vi "COPY_DLL_TO_C.vi"(8 "error in (no error)":errorcluster, 10 "appended path in":path) -> (0 "error out":errorcluster, 2 "appended path out":path)   [LabVIEW 2015, in "VIS-NIR.lvclass"]
uses:
  VIS-IR/VIS-NIR.lvclass
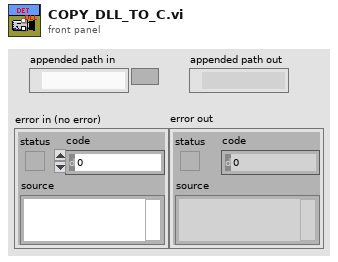
[diagram p1: front panel]
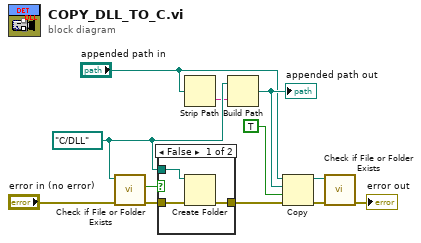
[diagram p0: block diagram]
diagram:
  w10 = path "C:/DLL" ("appended path")
  n1 = call <vilib>:"Check if File or Folder Exists.vi"("error in (no error)"="error in (no error)", "path"=w10) -> ("error out"=w9:errorcluster, "file or folder exists?"=w7:bool)  [unwired: 7 in, 1 out]
  n2 = case shown="False" w7 {
    tunnel: [w13 w16] -> w8
    tunnel: w9 -> [w14 w16]
    tunnel: w10 -> [w15 _]
    frame False {
      n3 = Create Folder(path (use dialog)=w15, error in=w14) -> (error out=w13:errorcluster)  [unwired: 1 in, 2 out]
    }
    frame True {
    }
  }
  n4 = Strip Path(path="appended path in") -> (name=w3:string)  [unwired: 1 out]
  n5 = Build Path(base path=w10, name or relative path=w3) -> (appended path=w12:path)
  "appended path out" <- w12
  n6 = Copy(8:w8, 9:TRUE ("overwrite (F)"), 10:w12, 11:"appended path in") -> (0:w5:errorcluster, 3:w4:path)  [unwired: 1 in, 1 out]
  n7 = call <vilib>:"Check if File or Folder Exists.vi"("error in (no error)"=w5, "path"=w4) -> ("error out"=→"error out":errorcluster)  [unwired: 7 in, 2 out]
